vi "TcpReaderProcess.vi"(8 "error in (no error)":errorcluster, 10 "Pound":refnum<class "Pound.lvclass">, 11 "Qbus in":refnum<class "Qbus.lvclass">) -> (0 "error out":errorcluster)   [LabVIEW 2017, in "ServerComm.lvlib"]
uses:
  <vilib>/addons/InsightCM/Devices/Shared/Common/ServerComm/ServerComm.lvlib
  <vilib>/addons/Qbus/Qbus.lvclass
  <vilib>/NI/Software Watchdog/Pound/Pound.lvclass
  <vilib>/addons/InsightCM/Devices/Shared/Common/ServerComm/controls/TcpReaderConfig.ctl
  <vilib>/addons/InsightCM/MessageBus/TcpApi/controls/TcpMessageReference.ctl
  <vilib>/addons/InsightCM/Devices/Shared/Common/ServerComm/controls/ConnectedStatusDvr.ctl
  <vilib>/addons/InsightCM/Devices/Shared/Common/ServerComm/controls/ConnectionStatus.ctl
  <vilib>/addons/TraceLogger/TraceLogger.lvlib
  <vilib>/NI/Software Watchdog/Watchdog/Watchdog.lvclass
  <vilib>/addons/InsightCM/Utilities/GlobalConfiguration/GlobalConfiguration.lvlib
  <vilib>/addons/InsightCM/Utilities/PropertyHelpers/PropertyHelpers.lvlib
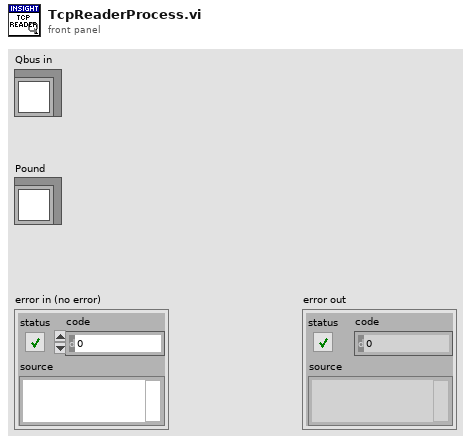
[diagram p1: front panel]
types:
  T1 = typedef "ServerComm.lvlib/TcpReaderConfig.ctl" = cluster{"tcp reference":T2, "connected":T3}
  T2 = typedef "TcpMessageReference.ctl" = refnum<data-value>
  T3 = typedef "ServerComm.lvlib/ConnectedStatusDvr.ctl" = refnum<data-value>
  T4 = typedef "SectionKeyValues.ctl" = cluster{"Section":string, "KeyValues":T5[]}
  T5 = typedef "KeyValuePair.ctl" = cluster{"Key":string, "Value":string}
  T6 = typedef "ServerComm.lvlib/ConnectionStatus.ctl" = enum16{"Offline", "NotAuthorized", "Online"}
  T7 = typedef "Message.ctl" = cluster{"Header":T8, "Body":u8[]}
  T8 = typedef "MessageHeader.ctl" = cluster{"MessageName":string, "Timestamp":i64, "CorrelationId":string, "ContentType":string, "RoutingKey":string, "Properties":T5[]}
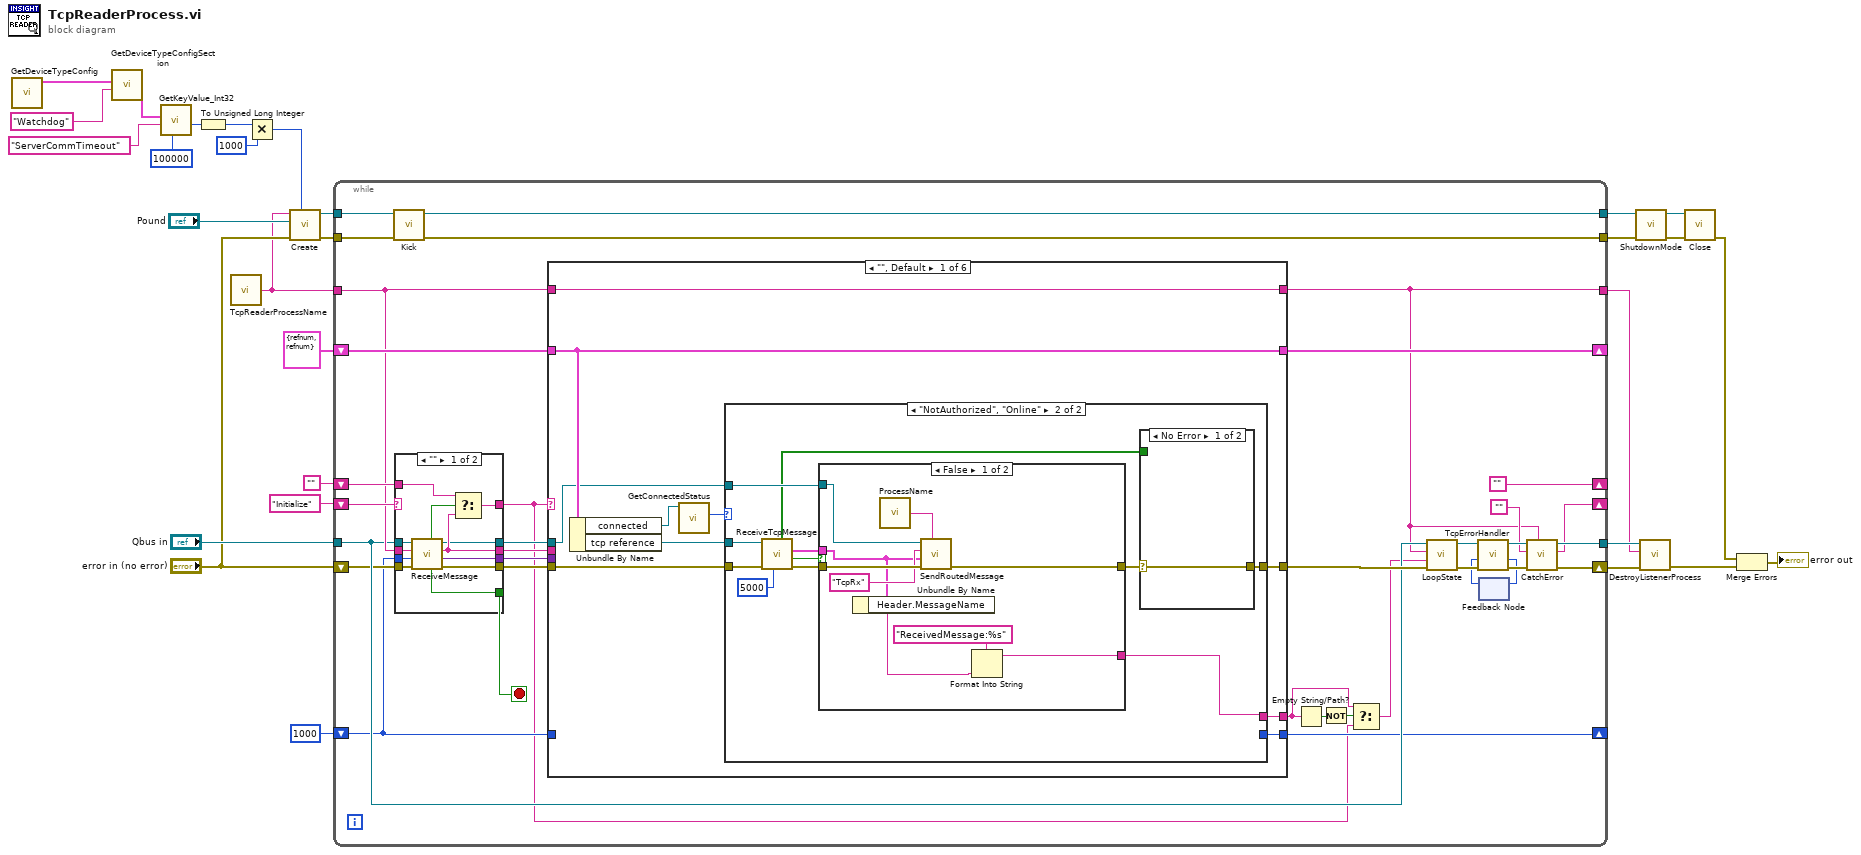
[diagram p0: block diagram]
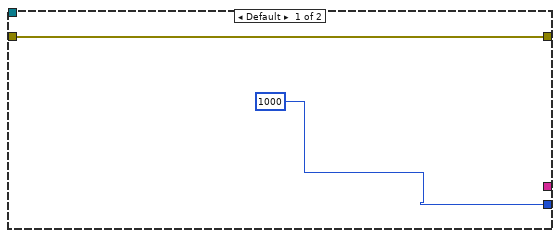
[diagram p3: hidden frame]
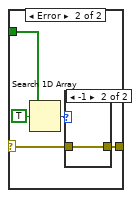
[diagram p4: hidden frame]
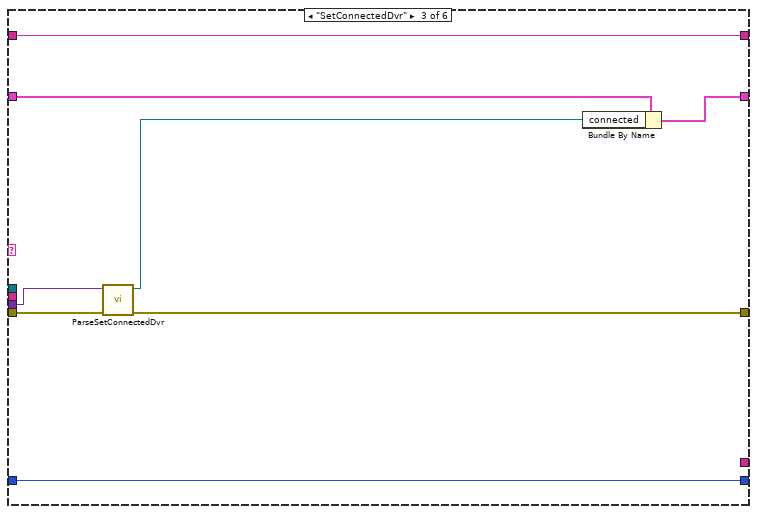
[diagram p8: hidden frame]
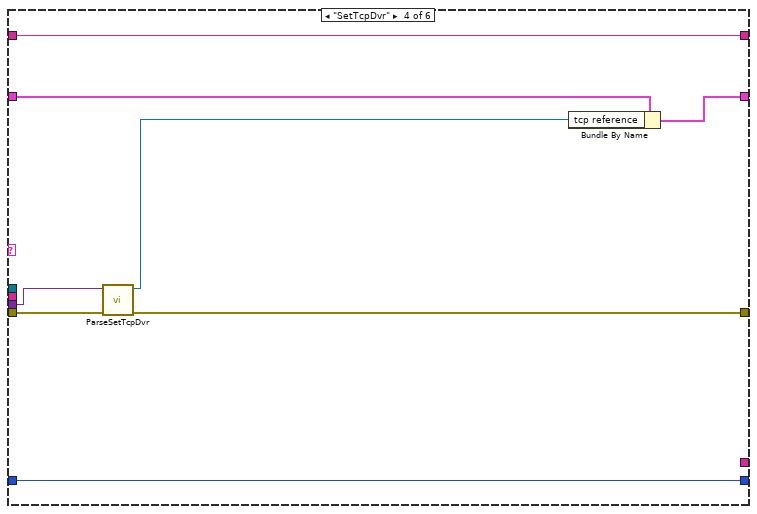
[diagram p9: hidden frame]
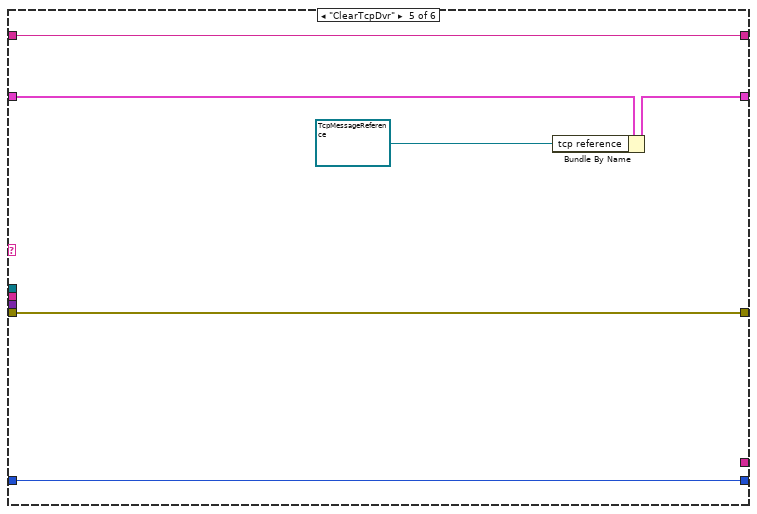
[diagram p10: hidden frame]
diagram:
  n1 = call <vilib>:"GetDeviceTypeConfig.vi"() -> ("key values"=w9:T4[])  [unwired: 9 in, 2 out]
  n2 = call <vilib>:"GetDeviceTypeConfigSection.vi"("key"="Watchdog", "key values"=w9) -> ("key value pairs out"=w7:T5[])  [unwired: 8 in, 1 out]
  n3 = call <vilib>:"GetKeyValue_Int32.vi"("default"=100000 ("Execution Timeout (ms)"), "key"="ServerCommTimeout" ("Tag"), "key value pairs"=w7) -> ("value"=w5:i32)  [unwired: 6 in, 2 out]
  n4 = To Unsigned Long Integer(number=w5) -> (unsigned 32bit integer=w2:u32)
  n5 = call <vilib>:"TcpReaderProcessName.vi"() -> ("process name"=w13:string)  [unwired: 5 in]
  n6 = Multiply(x=w2, y=u32 1000) -> (x*y=w1:u32)
  n7 = call <vilib>:"Create.vi"("Execution Timeout (ms)"=w1, "error in (no error)"="error in (no error)", "Pound"="Pound", "Name"=w13) -> ("error out"=w18:errorcluster, "Watchdog"=w19:refnum<data-value>)  [unwired: 6 in]
  n8 = while {
    shift-right: [""] -> _
    shift-left: "" -> [w64]
    tunnel: "Qbus in" -> [w47]
    tunnel: w13 -> [w48]
    tunnel: [w53] -> w27
    tunnel: [w37] -> w26
    shift-right: [w51] -> _
    shift-left: "Initialize" -> [w58]
    shift-right: [w44] -> _
    shift-left: T1 {"tcp reference"=refnum, "connected"=refnum} ("config") -> [w57]
    shift-right: [w43] -> _
    shift-left: 1000 ("milliseconds to wait") -> [w42]
    tunnel: w19 -> [w41]
    tunnel: w18 -> [w40]
    tunnel: [w39] -> w17
    tunnel: [w38] -> w16
    shift-right: [w55] -> w28
    shift-left: "error in (no error)" -> [w45]
    stop <- w65 stop-if-true
    n9 = call <vilib>:"Kick.vi"("error in (no error)"=w40, "Watchdog"=w41) -> ("error out"=w38:errorcluster, "Watchdog"=w39:refnum<data-value>)  [unwired: 8 in]
    n10 = case shown="\"\"" w58 {
      selector: w58 -> [_ w78]
      tunnel: w45 -> [w68 w80]
      tunnel: [w74 w80] -> w63
      tunnel: [w73 _] -> w59
      tunnel: [w69 _] -> w65
      tunnel: [w72 _] -> w60
      tunnel: w64 -> [w77 _]
      tunnel: [w76 w78] -> w31
      tunnel: [w71 w79] -> w61
      tunnel: w42 -> [w67 _]
      tunnel: w47 -> [w70 w79]
      tunnel: w48 -> [w66 _]
      frame "" {
        n11 = call <vilib>:"ReceiveMessage.vi"("error in (no error)"=w68, "timeout (0)"=w67, "process name"=w66, "Qbus in"=w70) -> ("error in (no error)"=w74:errorcluster, "message value"=w73:variant, "message name"=w72:string, "Qbus out"=w71:refnum<class "Qbus.lvclass">, "exit"=w69:bool, "timed out"=w75:bool)  [unwired: 2 in]
        n12 = Select(t=w77, s=w75, f=w72) -> (s? t:f=w76:string)
      }
      frame Default {
      }
    }
    n13 = case shown="\"\", Default" w31 {
      tunnel: w63 -> [w87 w121 w132 w140 w143 w147]
      tunnel: w61 -> [w84 _ _ _ _ _]
      tunnel: [w85 w121 w131 w139 w143 w147] -> w50
      tunnel: w60 -> [_ _ _ _ _ _]
      tunnel: w59 -> [_ _ w130 w138 _ _]
      tunnel: w57 -> [w86 w124 w129 w137 w146 w150]
      tunnel: [w86 w124 w128 w136 w145 w150] -> w44
      tunnel: w48 -> [w82 w122 w125 w133 w141 w149]
      tunnel: [w83 w123 w126 w134 w144 w148] -> w43
      tunnel: w42 -> [_ w123 w126 w134 w144 w148]
      tunnel: [w82 w122 w125 w133 w141 w149] -> w37
      tunnel: [w81 _ _ _ _ _] -> w32
      frame "", Default {
        n14 = Unbundle By Name(w86) -> ("connected"=w89:T3, "tcp reference"=w88:T2)
        n15 = call <vilib>:"GetConnectedStatus.vi"("dvr connected"=w89) -> ("status"=w90:T6)  [unwired: 5 in, 1 out]
        n16 = case shown="\"NotAuthorized\", \"Online\"" w90 {
          tunnel: w87 -> [w92 w103]
          tunnel: w88 -> [_ w99]
          tunnel: [w92 w95] -> w85
          tunnel: w84 -> [_ w97]
          tunnel: [1000 ("milliseconds to wait") _] -> w83
          tunnel: [_ w93] -> w81
          frame Default {
          }
          frame "NotAuthorized", "Online" {
            n17 = call <vilib>:"ReceiveTcpMessage.vi"("timeout (5 sec)"=5000, "error in (no error)"=w103, "connection ID in"=w99) -> ("error out"=w101:errorcluster, "timed out"=w102:bool, "message"=w100:T7, "ByteReadErrors"=w94:bool[])  [unwired: 3 in, 2 out]
            n18 = case shown="False" w102 {
              tunnel: w101 -> [w117 w120]
              tunnel: w97 -> [w119 _]
              tunnel: w100 -> [w114 _]
              tunnel: [w118 w120] -> w96
              tunnel: [w111 _] -> w93
              frame False {
                n19 = Unbundle By Name(w114) -> ("Header.MessageName"=w112:string)
                n20 = call <vilib>:"ProcessName.vi"() -> ("process name"=w115:string)  [unwired: 5 in]
                n21 = call <vilib>:"SendRoutedMessage.vi"("listener process"=w115, "error in (no error)"=w117, "message value"=w114, "message name"="TcpRx" ("MsgName"), "Qbus in"=w119) -> ("error in (no error)"=w118:errorcluster)  [unwired: 5 in, 1 out]
                n22 = Format Into String(format string="ReceivedMessage:%s", w112) -> (resulting string=w111:string)  [unwired: 2 in, 1 out]
              }
              frame True {
              }
            }
            n23 = case shown="No Error" w96 {
              selector: w96 -> [w104 w106]
              tunnel: [w104 w105] -> w95
              tunnel: w94 -> [_ w109]
              frame No Error {
              }
              frame Error {
                n24 = Search 1D Array(1D array=w109, element=TRUE) -> (index of element=w107:i32)  [unwired: 1 in]
                n25 = case shown="-1" w107 {
                  tunnel: w106 -> [_ w110]
                  tunnel: [_ w110] -> w105
                  frame 0, Default {
                  }
                  frame -1 {
                  }
                }
              }
            }
          }
        }
      }
      frame "Initialize" {
      }
      frame "SetConnectedDvr" {
        n26 = call <vilib>:"ParseSetConnectedDvr.vi"("error in (no error)"=w132, "body"=w130) -> ("error out"=w131:errorcluster, "connected"=w127:T3)  [unwired: 8 in]
        n27 = Bundle By Name(cluster=w129, "connected"=w127) -> (w128:T1)
      }
      frame "SetTcpDvr" {
        n28 = call <vilib>:"ParseSetTcpDvr.vi"("error in (no error)"=w140, "body"=w138) -> ("error out"=w139:errorcluster, "tcp reference"=w135:T2)  [unwired: 8 in]
        n29 = Bundle By Name(cluster=w137, "tcp reference"=w135) -> (w136:T1)
      }
      frame "ClearTcpDvr" {
        n30 = Bundle By Name(cluster=w146, "tcp reference"=T2 refnum) -> (w145:T1)
      }
      frame "Exit" {
      }
    }
    n31 = Empty String/Path?(string/path=w32) -> (empty?=w34:bool)
    n32 = Not(x=w34) -> (.not. x?=w33:bool)
    n33 = Select(t=w32, s=w33, f=w31) -> (s? t:f=w30:string)
    n34 = call <vilib>:"LoopState.vi"("error in (no error)"=w50, "loop action"=w30, "process name"=w37, "Qbus in"=w47) -> ("error out"=w49:errorcluster, "Qbus out"=w46:refnum<class "Qbus.lvclass">)  [unwired: 6 in]
    n35 = feedback #1() -> (w35:i32)  [unwired: 1 in]
    n36 = call <vilib>:"TcpErrorHandler.vi"("error in (no error)"=w49, "consequtive error count in"=w35, "Qbus in"=w46) -> ("error out"=w56:errorcluster, "consequtive error count out"=w36:i32, "Qbus out"=w54:refnum<class "Qbus.lvclass">)  [unwired: 6 in]
    n37 = feedback-in #1(w36) -> ()
    n38 = call <vilib>:"CatchError.vi"("source"=w37, "error in (no error)"=w56, "next action in"="", "Qbus in"=w54) -> ("error out"=w55:errorcluster, "next action out"=w51:string, "Qbus out"=w53:refnum<class "Qbus.lvclass">)  [unwired: 5 in]
  }
  n39 = call <vilib>:"ShutdownMode.vi"("error in (no error)"=w16, "Watchdog"=w17) -> ("error out"=w20:errorcluster, "Watchdog"=w21:refnum<data-value>)  [unwired: 8 in]
  n40 = call <vilib>:"DestroyListenerProcess.vi"("error in (no error)"=w28, "process name"=w26, "Qbus in"=w27) -> ("error in (no error)"=w11:errorcluster)  [unwired: 7 in, 1 out]
  n41 = call <vilib>:"Close.vi"("error in (no error)"=w20, "Watchdog"=w21) -> ("error out"=w12:errorcluster)  [unwired: 9 in]
  n42 = Merge Errors(w12, w11) -> (→"error out":errorcluster)
